vi "Get Listbox FocusRow Text.vi"(8 "error in (no error)":errorcluster, 11 "LstBox Refnum":refnum<vi>) -> (0 "error out":errorcluster, 1 "Selected Index":i32, 2 "Selected Item":string, 3 "Listbox Ref out":refnum<vi>)   [LabVIEW 2015]
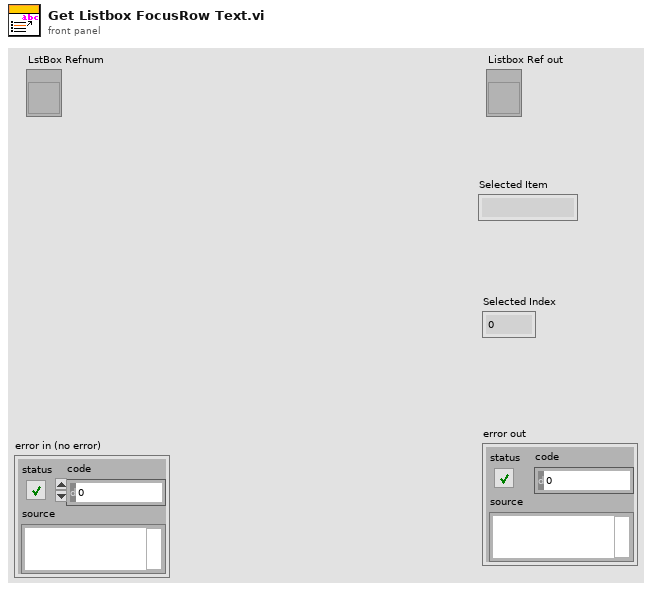
[diagram p1: front panel]
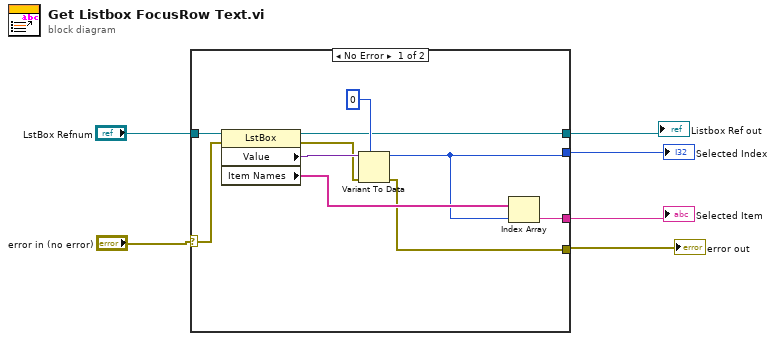
[diagram p0: block diagram]
diagram:
  n1 = case shown="No Error" "error in (no error)" {
    selector: "error in (no error)" -> [w9 w18]
    tunnel: [w15 _] -> w6
    tunnel: "LstBox Refnum" -> [w14 w17]
    tunnel: [w10 w17] -> w4
    tunnel: [w8 w18] -> w2
    tunnel: [w7 _] -> w1
    frame No Error {
      n2 = property class="LstBox"(reference=w14, error in=w9) -> (reference out=w10:refnum<vi>, error out=w12:errorcluster, "Value"=w13:variant, "Item Names"=w16:string[])
      n3 = Variant To Data(error in=w12, type=0, Variant=w13) -> (data=w7:i32, error out=w8:errorcluster)
      n4 = Index Array(array=w16, index=w7) -> (element=w15:string)
    }
    frame Error {
    }
  }
  "Selected Item" <- w6
  "Listbox Ref out" <- w4
  "error out" <- w2
  "Selected Index" <- w1
